vi "BRig_Host_comm_NetStream_testConnect.vi"() -> ()   [LabVIEW 2014]
panel:
  out "Waveform Chart":u16(graph)
  in  "stop":bool
  out "error out":errorcluster
  out "Listening":bool
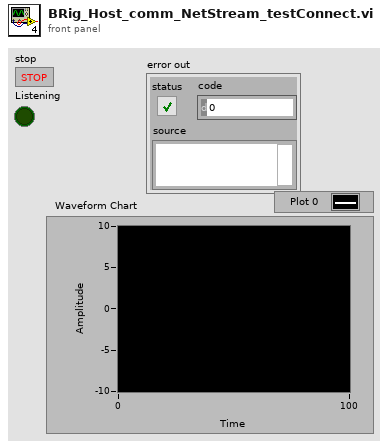
[diagram p1: front panel]
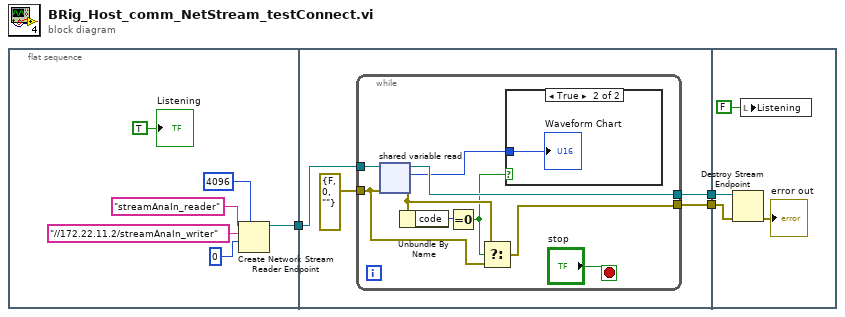
[diagram p0: block diagram]
diagram:
  n1 = flat-sequence {
    tunnel: [w4] -> w3
    tunnel: w3 -> [w13]
    tunnel: [w11] -> w2
    tunnel: [w10] -> w1
    tunnel: w2 -> [w25]
    tunnel: w1 -> [w24]
    frame #0 {
      n2 = Create Network Stream Reader Endpoint(7:4096 ("reader buffer size"), 9:u16 0 ("element"), 10:"//172.22.11.2/streamAnaIn_writer" ("writer url"), 11:"streamAnaIn_reader" ("reader name")) -> (3:w4:refnum<k21>)  [unwired: 3 in, 1 out]
      "Listening" <- TRUE ("Listening")
    }
    frame #1 {
      n3 = while {
        tunnel: w13 -> [w21]
        tunnel: errorcluster {"status"=FALSE, "code"=0, "source"=""} ("error in (no error)") -> [w18]
        tunnel: [w17] -> w11
        tunnel: [w16] -> w10
        stop <- "stop" stop-if-true
        n4 = shared-variable-read(w21, w18) -> (w17:refnum<k21>, w19:errorcluster, w14:u16)  [unwired: 1 in, 1 out]
        n5 = Unbundle By Name(w19) -> ("code"=w22:i32)
        n6 = Equal To 0?(x=w22) -> (x = 0?=w15:bool)
        n7 = Select(t=w19, s=w15, f=w18) -> (s? t:f=w16:errorcluster)
        n8 = case shown="True" w15 {
          tunnel: w14 -> [_ w23]
          frame False {
          }
          frame True {
            "Waveform Chart" <- w23
          }
        }
      }
    }
    frame #2 {
      n9 = Destroy Stream Endpoint(8:w24, 11:w25) -> (0:→"error out":errorcluster)
      n10 = local write "Listening"(FALSE ("Listening")) -> ()
    }
  }
